vi "Connect with Connection Cluster.vi"(8 "error in (no error)":errorcluster, 10 "Connection Info":T1, 11 "object in":refnum<class "JuPyter_Client.lvclass">) -> (0 "error out":errorcluster, 3 "object out":refnum<class "JuPyter_Client.lvclass">)   [LabVIEW 2018, in "JuPyter_Client.lvclass"]
doc: "Connect to an existing kernel"
uses:
  JuPyter_Client.lvclass
  Utility/Connection.ctl
  JuPyter_Client.lvclass/JuPyter_Client.ctl
  <vilib>/addons/zeromq/socket_type.ctl
  <vilib>/addons/zeromq/socket_options.ctl
  <vilib>/addons/zeromq/zmq_socket.lvclass
  <vilib>/addons/zeromq/zmq_context.lvclass
  <vilib>/addons/zeromq/zeromq.lvlib
  ClientMessaging.lvlib
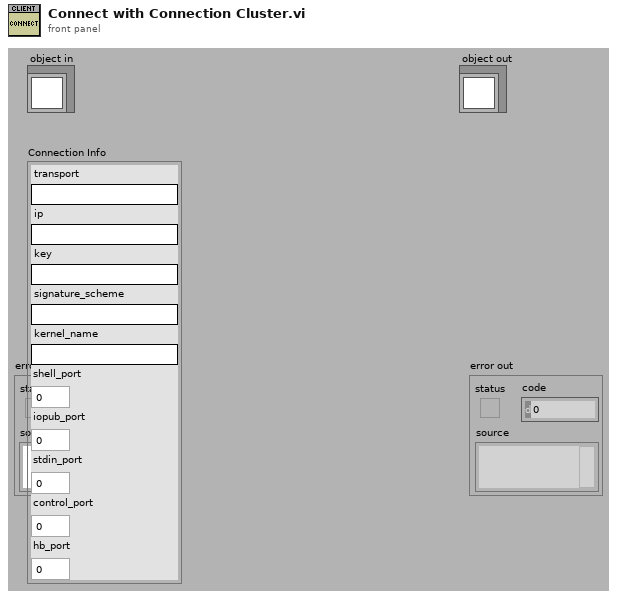
[diagram p1: front panel]
types:
  T1 = typedef "ClientMessaging.lvlib/Connection.ctl" = cluster{"transport":string, "ip":string, "key":string, "signature_scheme":string, "kernel_name":string, "shell_port":u16, "iopub_port":u16, "stdin_port":u16, "control_port":u16, "hb_port":u16}
  T2 = enum16{"Shell", "IOPub", "Stdin", "Control", "Heart Beat"}
  T3 = typedef "zeromq.lvlib/socket_type.ctl" = enum8{"ZMQ_PAIR", "ZMQ_PUB", "ZMQ_SUB", "ZMQ_REQ", "ZMQ_REP", "ZMQ_DEALER", "ZMQ_ROUTER", "ZMQ_PULL", "ZMQ_PUSH", "ZMQ_XPUB", "ZMQ_XSUB"}
  T4 = typedef "zeromq.lvlib/socket_options.ctl" = enum8{"NONE", "ZMQ_HWM", "<2>", "ZMQ_SWAP", "ZMQ_AFFINITY", "ZMQ_IDENTITY", "ZMQ_SUBSCRIBE", "ZMQ_UNSUBSCRIBE", "ZMQ_RATE", "ZMQ_RECOVERY_IVL", "ZMQ_MCAST_LOOP", "ZMQ_SNDBUF", "ZMQ_RCVBUF", "ZMQ_RCVMORE", "ZMQ_FD", "ZMQ_EVENTS", "ZMQ_TYPE", "ZMQ_LINGER", "ZMQ_RECONNECT_IVL", "ZMQ_BACKLOG", "ZMQ_RECOVERY_IVL_MSEC", "ZMQ_RECONNECT_IVL_MAX", "ZMQ_MAXMSGSIZE", "ZMQ_SNDHWM", "ZMQ_RCVHWM", "ZMQ_MULTICAST_HOPS", "<26>", "ZMQ_RCVTIMEO", "ZMQ_SNDTIMEO", "<29>", "<30>", "ZMQ_IPV4ONLY", "ZMQ_LAST_ENDPOINT", "ZMQ_ROUTER_MANDATORY", "ZMQ_TCP_KEEPALIVE", "ZMQ_TCP_KEEPALIVE_CNT", "ZMQ_TCP_KEEPALIVE_IDLE", "ZMQ_TCP_KEEPALIVE_INTVL", "ZMQ_TCP_ACCEPT_FILTER", "ZMQ_DELAY_ATTACH_ON_CONNECT", "ZMQ_XPUB_VERBOSE"}
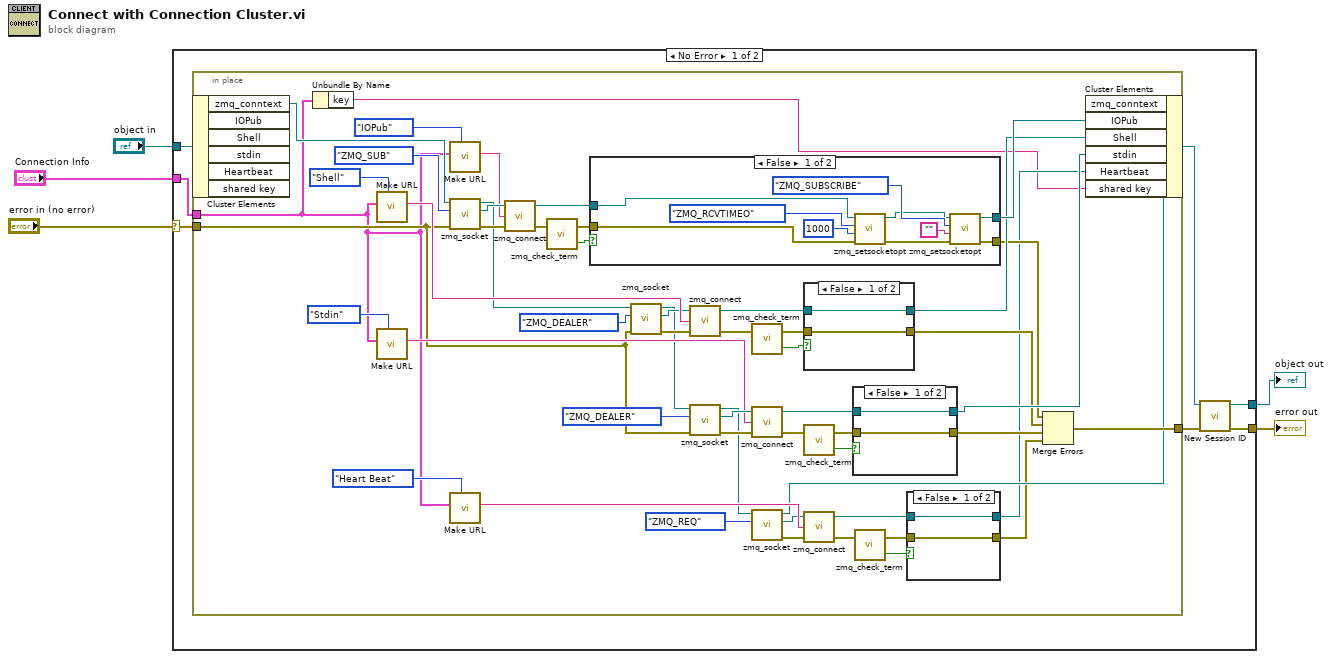
[diagram p0: block diagram]
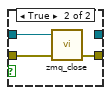
[diagram p2: hidden frame]
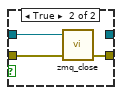
[diagram p3: hidden frame]
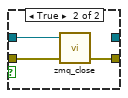
[diagram p4: hidden frame]
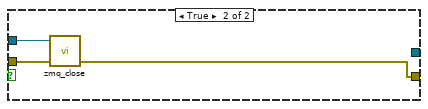
[diagram p5: hidden frame]
diagram:
  n1 = case shown="No Error" "error in (no error)" {
    selector: "error in (no error)" -> [w6 w95]
    tunnel: [w8 w95] -> w4
    tunnel: [w10 w94] -> w2
    tunnel: "object in" -> [w12 w94]
    tunnel: "Connection Info" -> [w7 _]
    frame No Error {
      n2 = in-place {
        in-place-border: w7 -> [w14]
        in-place-border: w6 -> [w34]
        in-place-border: [w28] -> w9
        n3 = in-place-cluster #1(w12) -> ("zmq_conntext"=w65:refnum<class "zmq_context.lvclass">)  [unwired: 5 out]
        n4 = Unbundle By Name(w14) -> ("key"=w13:string)
        n5 = call "Make URL.vi"("Port"=T2."Shell", "Connection Info"=w14) -> ("Connection URL"=w50:string)  [unwired: 9 in]
        n6 = call "Make URL.vi"("Port"=T2."Stdin", "Connection Info"=w14) -> ("Connection URL"=w45:string)  [unwired: 9 in]
        n7 = call "Make URL.vi"("Port"=T2."IOPub", "Connection Info"=w14) -> ("Connection URL"=w62:string)  [unwired: 9 in]
        n8 = call <vilib>:"zmq_socket.vi"("error in"=w34, "socket type"=socket_type."ZMQ_SUB", "context in"=w65) -> ("error out"=w61:errorcluster, "socket out"=w63:refnum<class "zmq_socket.lvclass">, "context out"=w39:refnum<class "zmq_context.lvclass">)  [unwired: 2 in]
        n9 = call "Make URL.vi"("Port"=T2."Heart Beat", "Connection Info"=w14) -> ("Connection URL"=w21:string)  [unwired: 9 in]
        n10 = call <vilib>:"zmq_connect.vi"("error in"=w61, "endpoint"=w62, "socket in"=w63) -> ("error out"=w60:errorcluster, "socket out"=w58:refnum<class "zmq_socket.lvclass">)  [unwired: 1 in]
        n11 = call <vilib>:"zmq_check_term.vi"("error in"=w60) -> ("term?"=w59:bool, "error out"=w57:errorcluster)  [unwired: 1 in]
        n12 = case shown="False" w59 {
          tunnel: w58 -> [w85 w93]
          tunnel: w57 -> [w86 w92]
          tunnel: [w88 w91] -> w31
          tunnel: [w90 _] -> w56
          frame False {
            n13 = call <vilib>:"zmq_setsocketopt.vi"("error in"=w86, "value"=1000, "option"=socket_options."ZMQ_RCVTIMEO", "socket in"=w85) -> ("error out"=w84:errorcluster, "socket out"=w83:refnum<class "zmq_socket.lvclass">)  [unwired: 2 in]
            n14 = call <vilib>:"zmq_setsocketopt.vi"("error in"=w84, "value"="", "option"=socket_options."ZMQ_SUBSCRIBE", "socket in"=w83) -> ("error out"=w88:errorcluster, "socket out"=w90:refnum<class "zmq_socket.lvclass">)  [unwired: 2 in]
          }
          frame True {
            n15 = call <vilib>:"zmq_close.vi"("error in"=w92, "socket"=w93) -> ("error out"=w91:errorcluster)  [unwired: 3 in]
          }
        }
        n16 = call <vilib>:"zmq_socket.vi"("error in"=w34, "socket type"=socket_type."ZMQ_DEALER", "context in"=w39) -> ("error out"=w51:errorcluster, "socket out"=w49:refnum<class "zmq_socket.lvclass">, "context out"=w38:refnum<class "zmq_context.lvclass">)  [unwired: 2 in]
        n17 = call <vilib>:"zmq_connect.vi"("error in"=w51, "endpoint"=w50, "socket in"=w49) -> ("error out"=w52:errorcluster, "socket out"=w54:refnum<class "zmq_socket.lvclass">)  [unwired: 1 in]
        n18 = call <vilib>:"zmq_socket.vi"("error in"=w34, "socket type"=socket_type."ZMQ_DEALER", "context in"=w38) -> ("error out"=w44:errorcluster, "socket out"=w46:refnum<class "zmq_socket.lvclass">, "context out"=w18:refnum<class "zmq_context.lvclass">)  [unwired: 2 in]
        n19 = call <vilib>:"zmq_check_term.vi"("error in"=w52) -> ("term?"=w53:bool, "error out"=w55:errorcluster)  [unwired: 1 in]
        n20 = call <vilib>:"zmq_connect.vi"("error in"=w44, "endpoint"=w45, "socket in"=w46) -> ("error out"=w43:errorcluster, "socket out"=w41:refnum<class "zmq_socket.lvclass">)  [unwired: 1 in]
        n21 = call <vilib>:"zmq_socket.vi"("socket type"=socket_type."ZMQ_REQ", "context in"=w18) -> ("error out"=w22:errorcluster, "socket out"=w20:refnum<class "zmq_socket.lvclass">, "context out"=w17:refnum<class "zmq_context.lvclass">)  [unwired: 3 in]
        n22 = case shown="False" w53 {
          tunnel: w54 -> [w76 w80]
          tunnel: w55 -> [w77 w79]
          tunnel: [w77 w78] -> w30
          tunnel: [w76 _] -> w33
          frame False {
          }
          frame True {
            n23 = call <vilib>:"zmq_close.vi"("error in"=w79, "socket"=w80) -> ("error out"=w78:errorcluster)  [unwired: 3 in]
          }
        }
        n24 = call <vilib>:"zmq_check_term.vi"("error in"=w43) -> ("term?"=w42:bool, "error out"=w40:errorcluster)  [unwired: 1 in]
        n25 = call <vilib>:"zmq_connect.vi"("error in"=w22, "endpoint"=w21, "socket in"=w20) -> ("error out"=w23:errorcluster, "socket out"=w25:refnum<class "zmq_socket.lvclass">)  [unwired: 1 in]
        n26 = case shown="False" w42 {
          tunnel: w41 -> [w71 w75]
          tunnel: w40 -> [w72 w74]
          tunnel: [w72 w73] -> w29
          tunnel: [w71 _] -> w32
          frame False {
          }
          frame True {
            n27 = call <vilib>:"zmq_close.vi"("error in"=w74, "socket"=w75) -> ("error out"=w73:errorcluster)  [unwired: 3 in]
          }
        }
        n28 = call <vilib>:"zmq_check_term.vi"("error in"=w23) -> ("term?"=w24:bool, "error out"=w26:errorcluster)  [unwired: 1 in]
        n29 = case shown="False" w24 {
          tunnel: w25 -> [w66 w70]
          tunnel: w26 -> [w67 w69]
          tunnel: [w67 w68] -> w15
          tunnel: [w66 _] -> w16
          frame False {
          }
          frame True {
            n30 = call <vilib>:"zmq_close.vi"("error in"=w69, "socket"=w70) -> ("error out"=w68:errorcluster)  [unwired: 3 in]
          }
        }
        n31 = Merge Errors(w31, w30, w29, w15) -> (w28:errorcluster)
        n32 = in-place-cluster #1("zmq_conntext"=w17, "IOPub"=w56, "Shell"=w33, "stdin"=w32, "Heartbeat"=w16, "shared key"=w13) -> (w11:refnum<class "JuPyter_Client.lvclass">)
      }
      n33 = call-dynamic "New Session ID.vi"("error in (no error)"=w9, "object in"=w11) -> ("error out"=w8:errorcluster, "object out"=w10:refnum<class "JuPyter_Client.lvclass">)  [unwired: 8 in]
    }
    frame Error {
    }
  }
  "error out" <- w4
  "object out" <- w2
